vi "FindNumberofMoves.vi"(11 "WayPointCluster":T1) -> (0 "max length":i32)   [LabVIEW 2023]
uses:
  TypeDefs/WayPointCluster.ctl
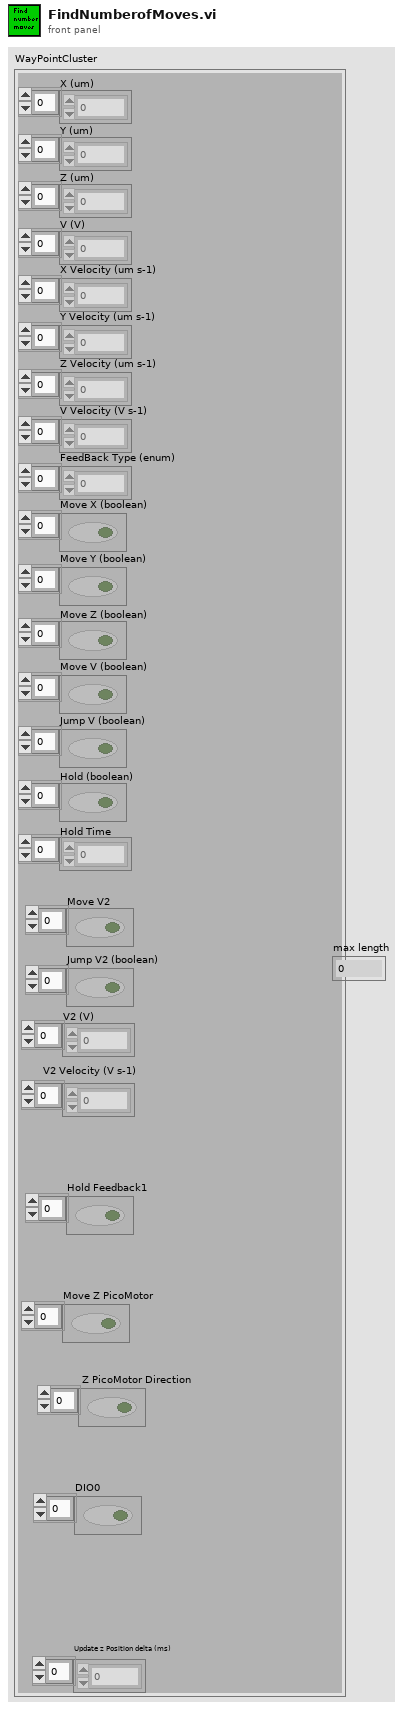
[diagram p1: front panel]
types:
  T1 = typedef "WayPointCluster.ctl" = cluster{"X (um)":dbl[], "Y (um)":dbl[], "Z (um)":dbl[], "V (V)":dbl[], "X Velocity (um s-1)":dbl[], "Y Velocity (um s-1)":dbl[], "Z Velocity (um s-1)":dbl[], "V Velocity (V s-1)":dbl[], "FeedBack Type (enum)":u16[], "Move X (boolean)":bool[], "Move Y (boolean)":bool[], "Move Z (boolean)":bool[], "Move V (boolean)":bool[], "Jump V (boolean)":bool[], "Hold (boolean)":bool[], "Hold Time":u32[], "V2 (V)":dbl[], "Move V2":bool[], "V2 Velocity (V s-1)":dbl[], "Jump V2 (boolean)":bool[], "Update z Position delta (ms)":i16[], "Hold Feedback1":bool[], "Move Z PicoMotor":bool[], " Z PicoMotor Direction":bool[], "DIO0":bool[]}
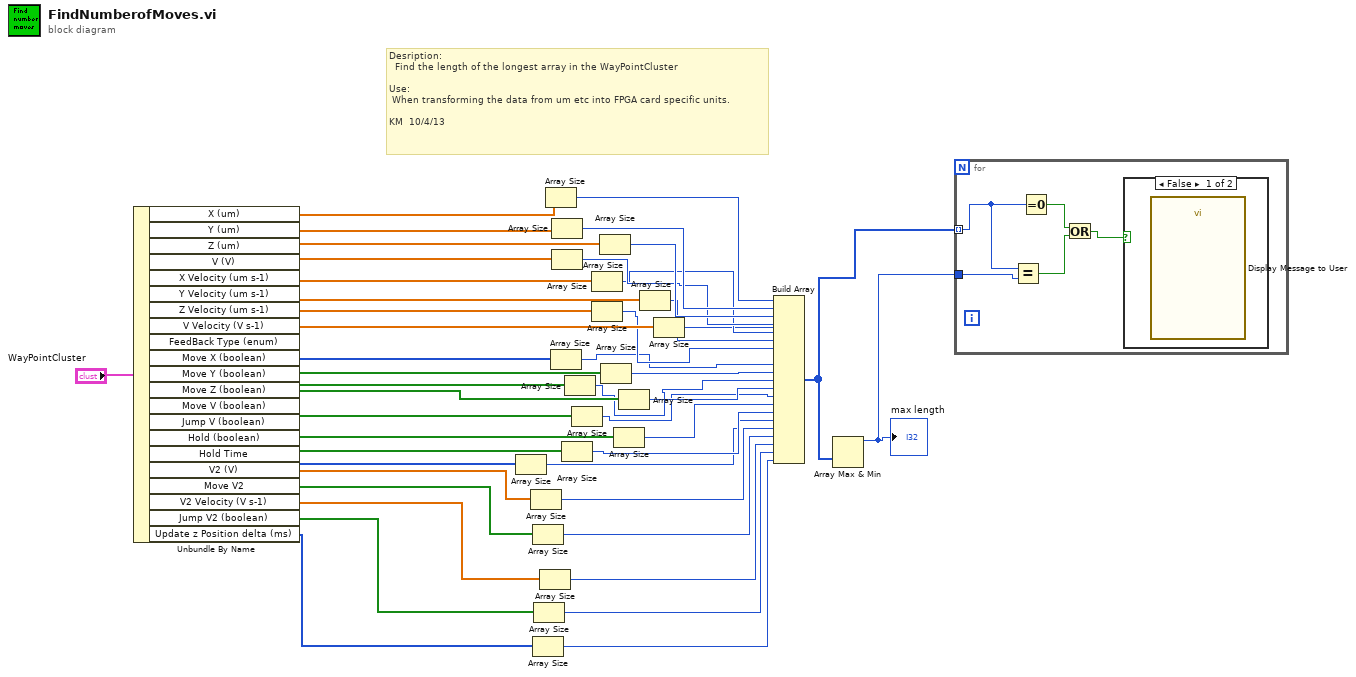
[diagram p0: block diagram]
diagram:
  # "Desription: \n  Find the length of the longest array in the WayPointCluster\n\nUse:\n When transforming the data from um etc into FPGA card specific units.\n\nKM  10/4/13"
  n1 = Unbundle By Name("WayPointCluster") -> ("X (um)"=w45:dbl[], "Y (um)"=w43:dbl[], "Z (um)"=w42:dbl[], "V (V)"=w41:dbl[], "X Velocity (um s-1)"=w40:dbl[], "Y Velocity (um s-1)"=w39:dbl[], "Z Velocity (um s-1)"=w38:dbl[], "V Velocity (V s-1)"=w37:dbl[], "FeedBack Type (enum)"=w36:u16[], "Move X (boolean)"=w35:bool[], "Move Y (boolean)"=w34:bool[], "Move Z (boolean)"=w33:bool[], "Move V (boolean)"=w32:bool[], "Jump V (boolean)"=w31:bool[], "Hold (boolean)"=w30:bool[], "Hold Time"=w29:u32[], "V2 (V)"=w12:dbl[], "Move V2"=w11:bool[], "V2 Velocity (V s-1)"=w10:dbl[], "Jump V2 (boolean)"=w9:bool[], "Update z Position delta (ms)"=w4:i16[])
  n2 = Array Size(array=w29) -> (size(s)=w13:i32)
  n3 = Array Size(array=w12) -> (size(s)=w8:i32)
  n4 = Array Size(array=w11) -> (size(s)=w7:i32)
  n5 = Array Size(array=w4) -> (size(s)=w3:i32)
  n6 = Array Size(array=w9) -> (size(s)=w5:i32)
  n7 = Array Size(array=w10) -> (size(s)=w6:i32)
  n8 = Array Size(array=w45) -> (size(s)=w28:i32)
  n9 = Array Size(array=w36) -> (size(s)=w20:i32)
  n10 = Array Size(array=w43) -> (size(s)=w27:i32)
  n11 = Array Size(array=w41) -> (size(s)=w25:i32)
  n12 = Array Size(array=w30) -> (size(s)=w14:i32)
  n13 = Array Size(array=w34) -> (size(s)=w18:i32)
  n14 = Array Size(array=w32) -> (size(s)=w16:i32)
  n15 = Array Size(array=w40) -> (size(s)=w24:i32)
  n16 = Array Size(array=w38) -> (size(s)=w22:i32)
  n17 = Array Size(array=w42) -> (size(s)=w26:i32)
  n18 = Array Size(array=w35) -> (size(s)=w19:i32)
  n19 = Array Size(array=w31) -> (size(s)=w15:i32)
  n20 = Array Size(array=w33) -> (size(s)=w17:i32)
  n21 = Array Size(array=w39) -> (size(s)=w23:i32)
  n22 = Array Size(array=w37) -> (size(s)=w21:i32)
  n23 = Build Array(w28, w27, w26, w25, w24, w23, w22, w21, w20, w19, w18, w17, w16, w15, w14, w13, w8, w7, w6, w5, w3) -> (w2:i32[])
  n24 = Array Max & Min(array=w2) -> (max value=w1:i32)  [unwired: 3 out]
  "max length" <- w1
  n25 = for {
    tunnel: w2 -> [w50] mode=indexing
    tunnel: w1 -> [w49]
    n26 = Equal?(x=w50, y=w49) -> (x = y?=w47:bool)
    n27 = Equal To 0?(x=w50) -> (x = 0?=w48:bool)
    n28 = Or(x=w48, y=w47) -> (x .or. y?=w46:bool)
    n29 = case shown="False" w46 {
      frame False {
        n30 = call "Display Message to User"() -> ()  [unwired: 10 in, 2 out]
      }
      frame True {
      }
    }
  }
